vi "Spreadsheet Storage (OpenWriteClose) (1).vi"() -> ()   [LabVIEW 2015]
panel:
  in  "Waveform Parameters":T1
  in  "Digitizing Parameters":T2
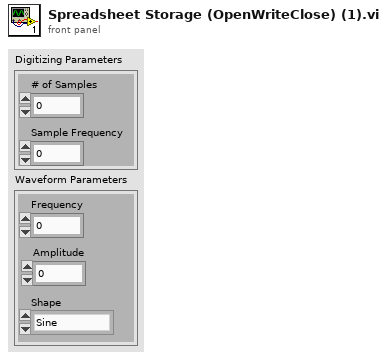
[diagram p1: front panel]
types:
  T1 = cluster{"Frequency":dbl, "Amplitude":dbl, "Shape":enum16{"Sine", "Cosine", "DC Level", "Square", "User-Defined"}}
  T2 = cluster{"# of Samples":i64, "Sample Frequency":dbl}
  T3 = enum16{"open", "replace", "create", "open or create", "replace or create", "replace or create with confirmation"}
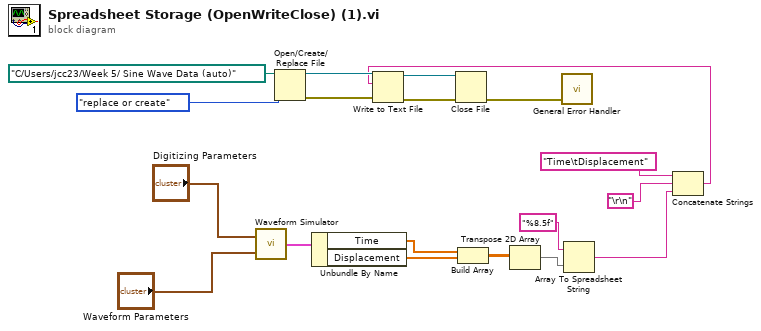
[diagram p0: block diagram]
diagram:
  n1 = call "Waveform Simulator.vi"("Waveform Parameters"="Waveform Parameters", "Digitizing Parameters"="Digitizing Parameters") -> ("Waveform Output"=w17:cluster{"Time":dbl[], "Displacement":dbl[]})
  n2 = Open/Create/Replace File(file path (use dialog)=path "C:/Users/jcc23/Week 5/ Sine Wave Data (auto)", operation (0:open)=T3."replace or create") -> (refnum out=w11:refnum<file>, error out=w14:errorcluster)  [unwired: 4 in, 1 out]
  n3 = Unbundle By Name(w17) -> ("Time"=w16:dbl[], "Displacement"=w15:dbl[])
  n4 = Build Array(w16, w15) -> (w8:dbl[][])
  n5 = Transpose 2D Array(2D array=w8) -> (transposed array=w7:dbl[][])
  n6 = Array To Spreadsheet String(array=w7, 3:"%8.5f" ("format string")) -> (spreadsheet string=w4:string)  [unwired: 1 in]
  n7 = Concatenate Strings("Time\tDisplacement" ("string"), "\r\n", w4) -> (w3:string)
  n8 = Write to Text File(file (use dialog)=w11, text=w3, error in=w14) -> (refnum out=w10:refnum<file>, error out=w13:errorcluster)  [unwired: 1 in, 1 out]
  n9 = Close File(refnum=w10, error in=w13) -> (error out=w12:errorcluster)  [unwired: 1 out]
  n10 = call <vilib>:"General Error Handler.vi"("error in (no error)"=w12) -> ()  [unwired: 10 in, 5 out]
